vi "read channel page lecroy.vi"(0 "VISA in":refnum<visa-resource-name>, 5 "Crate":i32, 7 "page":i32, 11 "error in":errorcluster) -> (4 "VISA out":refnum<visa-resource-name>, 6 "Array":T1[](array[typedef]) {"Vfile (V)" format="%.1f V"; "Vswmax (V)" format="%#_g V"; "Iset (A)" format="%.2pA"; "Imon (A)" format="%.2pA"; "Vset (V)" format="%#_g V"; "Vmon (V)" format="%.1f V"}, 8 "New Channels":T1[](array[typedef]) {"Vfile (V)" format="%.1f V"; "Vswmax (V)" format="%#_g V"; "Iset (A)" format="%.2pA"; "Imon (A)" format="%.2pA"; "Vset (V)" format="%#_g V"; "Vmon (V)" format="%.1f V"}, 10 "Start Index in ACTIVE":i32, 15 "error out":errorcluster)   [LabVIEW 2018]
uses:
  channel_cluster.ctl
  Tom Shaw/Lecroy Control/HV Documentation and Software for Testing/SubVIs/General_lecroy_command.ctl
  channel.ctl
  CAEN globals.vi
  <userlib>/_OpenG.lib/array/array.llb/Filter 1D Array with Scalar (I32)__ogtk.vi
panel:
  # "Press Ctrl+M to open the master for edit"
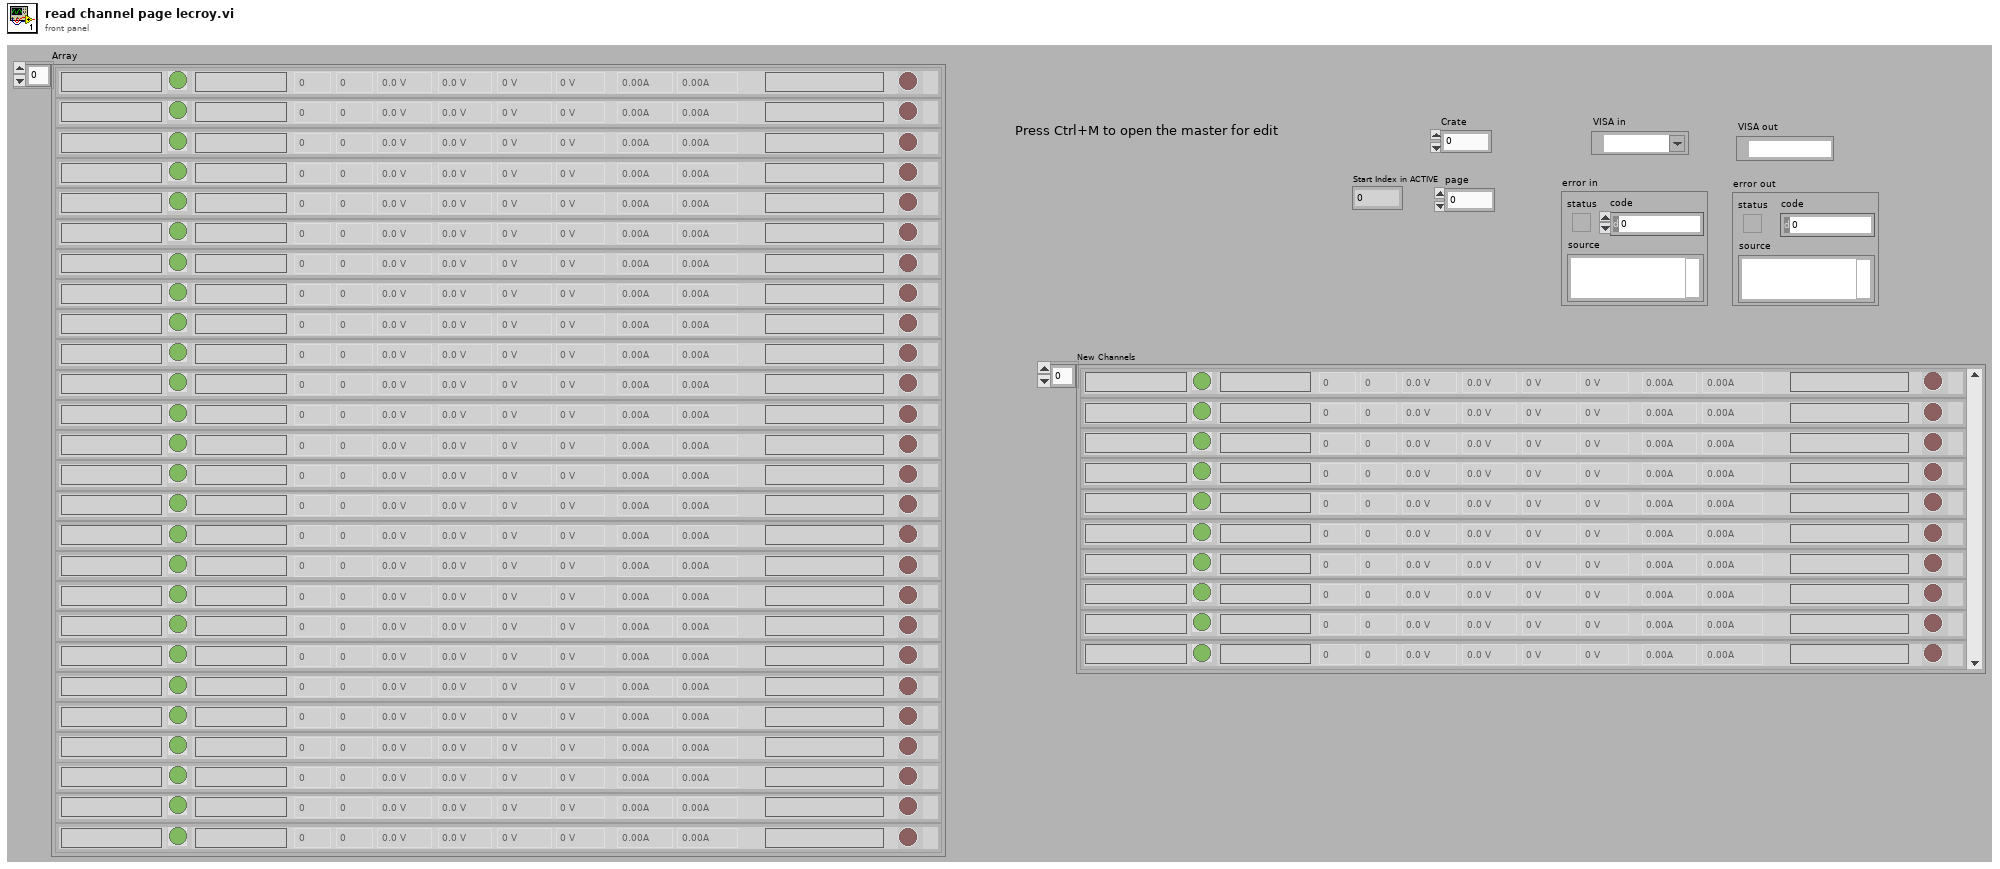
[diagram p1: front panel]
types:
  T1 = typedef "channel_cluster.ctl" = cluster{"Channel Name":string, "Crate":i32, "Card Type":string, "Card":i32, "Channel":i32, "Status Icon":picture, "Vmon (V)":dbl, "Vset (V)":dbl, "Imon (A)":dbl, "Iset (A)":dbl, "Timestamp":string, "ON/OFF":bool, "Status":string, "Vswmax (V)":dbl, "Flag":bool, "Vfile (V)":dbl, "Error Logged":bool[], "enable_file":bool}
  T2 = enum16{"Monitor", "Demand", "Backup", "All", "None"}
  T3 = typedef "crate.ctl" = cluster{"CAENet Address":i32, "Crate Model":string, "Firmware Version":string, "Crate Map":T4[], "Total Channels":i32}
  T4 = typedef "card.ctl" = cluster{"Slot Number":i32, "Card Model":string, "Num Channels":i32, "Polarity":string, "Vmax":dbl, "Imax":dbl, "Revision":string}
  T5 = typedef "General_lecroy_command.ctl" = string
  T6 = typedef "channel.ctl" = cluster{" Card.Channel":dbl, "Crate":i32}
  T7 = cluster{"Group Name":string, "Channels in Group":T6[]}[]
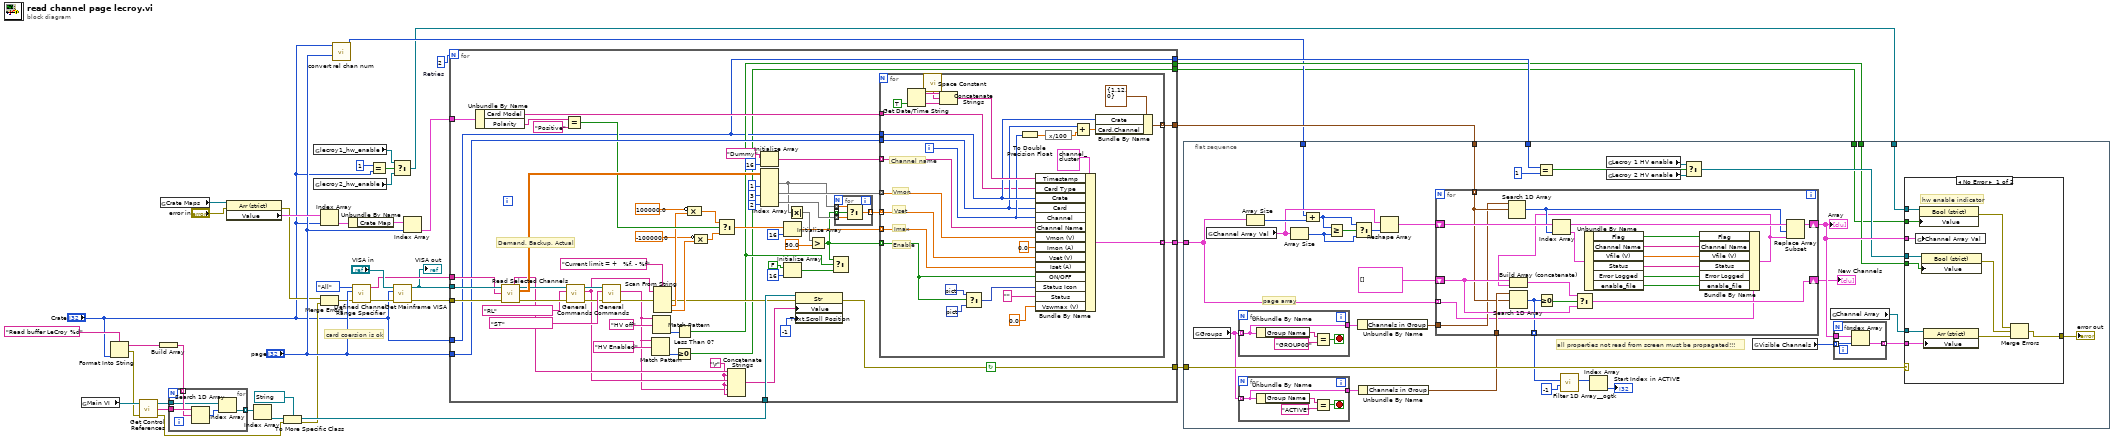
[diagram p0: block diagram]
diagram:
  w41 = 2  # Retries
  # "card coersion is ok"
  n1 = global read "CAEN globals.vi" "Main VI"() -> (w22:refnum<vi>)
  n2 = Format Into String(format string="Read buffer LeCroy %d" ("Label.Text"), "Crate") -> (resulting string=w12:string, error out=w13:errorcluster)  [unwired: 2 in]
  n3 = call "Get Control References.vi"("error in"=w13, "This vi"=w22) -> ("error out"=w19:errorcluster, "Control Names"=w23:string[], "Controls[]"=w24:refnum<vi>[])  [unwired: 1 in]
  n4 = Build Array(w12) -> (w14:string[])
  n5 = global read "CAEN globals.vi" "Crate Maps"() -> (w40:refnum<vi>)
  n6 = for {
    tunnel: w23 -> [w47]
    tunnel: w14 -> [w46] mode=indexing
    tunnel: w24 -> [w45]
    tunnel: [w44] -> w25 mode=indexing
    n7 = Search 1D Array(1D array=w47, element=w46) -> (index of element=w43:i32)  [unwired: 1 in]
    n8 = Index Array(array=w45, index=w43) -> (element=w44:refnum<vi>)
  }
  n9 = property class="Arr (strict)"(reference=w40, error in="error in") -> (error out=w17:errorcluster, "Value"=w30:T3[])  [unwired: 1 out]
  n10 = Index Array(array=w25) -> (element=w20:refnum<vi>)  [unwired: 1 in]
  n11 = To More Specific Class(target class=refnum<vi> refnum ("s? t:f"), reference=w20, error in=w19) -> (specific class reference=w18:refnum<vi>, error out=w16:errorcluster)
  n12 = global read "CAEN globals.vi" "lecroy1_hw_enable"() -> (w4:refnum<vi>)
  n13 = global read "CAEN globals.vi" "lecroy2_hw_enable"() -> (w3:refnum<vi>)
  n14 = Merge Errors(w17, w16) -> (w15:errorcluster)
  n15 = Index Array(array=w30, index="Crate") -> (element=w29:T3)
  n16 = call "convert rel chan num.vi"("Card"="page", "Crate"="Crate") -> ("Absolute index"=w8:i32)  [unwired: 6 in, 3 out]
  n17 = Unbundle By Name(w29) -> ("Crate Map"=w28:T4[])
  n18 = call "Defined Channel Range Specifier.vi"("error in"=w15, "Card"="page", "Buffer"=T2."All") -> ("error out"=w35:errorcluster, "Channel Range"=w34:string)  [unwired: 7 in]
  n19 = Equal?(x=1, y="Crate") -> (x = y?=w7:bool)
  n20 = Select(t=w4, s=w7, f=w3) -> (s? t:f=w2:refnum<vi>)
  n21 = call "Get Mainframe VISA.vi"("Error In"=w35, "Crate"="Crate", "VISA In"="VISA in") -> ("Error Out"=w37:errorcluster, "VISA out"=w32:refnum<visa-resource-name>)  [unwired: 6 in, 1 out]
  "VISA out" <- w32
  n22 = Index Array(array=w28, index="page") -> (element=w27:T4)
  n23 = for {
    N: w41 -> [_]
    tunnel: w32 -> [w106]
    tunnel: [w108] -> w31
    tunnel: w37 -> [w105]
    tunnel: [w61] -> w42
    tunnel: [w107] -> w39
    tunnel: w34 -> [w104]
    tunnel: "Crate" -> [w51]
    tunnel: "page" -> [w89]
    tunnel: w27 -> [w81]
    tunnel: w18 -> [w67]
    tunnel: [w56] -> w9
    tunnel: [w51] -> w10
    tunnel: [w50] -> w1
    stop <- w61 continue-if-true
    w63 = "\r"
    # "Demand, Backup, Actual"
    n24 = Unbundle By Name(w81) -> ("Card Model"=w87:string, "Polarity"=w86:string)
    n25 = call "Read Selected Channels.vi"("VISA in"=w106, "C##,##DO###"=w104, "error in"=w105) -> ("Final Output"=w66:string, "VISA out"=w98:refnum<visa-resource-name>, "Channel Array"=w103:dbl[][], "error out"=w99:errorcluster)  [unwired: 6 in, 3 out]
    n26 = Equal?(x=w86, y="Positive") -> (x = y?=w82:bool)
    n27 = call "General Commands.vi"("error in"=w99, "Action"=T5 "RL", "VISA in"=w98) -> ("error out"=w84:errorcluster, "result string"=w65:string, "VISA out"=w94:refnum<visa-resource-name>)  [unwired: 6 in]
    n28 = call "General Commands.vi"("error in"=w84, "Action"=T5 "ST", "VISA in"=w94) -> ("error out"=w83:errorcluster, "result string"=w48:string)  [unwired: 6 in, 1 out]
    n29 = Match Pattern(string=w48, regular expression="HV Enabled") -> (offset past match=w52:i32)  [unwired: 1 in, 3 out]
    n30 = Match Pattern(string=w48, regular expression="HV off") -> (offset past match=w78:i32)  [unwired: 1 in, 3 out]
    n31 = Scan From String(format string="Current limit = +   %f, - %f", input string=w65, error in=w83) -> (error out=w62:errorcluster, output 1=w74:dbl, output 2=w69:dbl)  [unwired: 3 in, 2 out]
    n32 = Greater Or Equal To 0?(x=w52) -> (x >= 0?=w50:bool)
    n33 = Less Than 0?(x=w78) -> (x < 0?=w56:bool)
    n34 = Compound Arithmetic op=MULTIPLY(invert 100000.0 ("value"), w74) -> (w73:dbl)
    n35 = Compound Arithmetic op=MULTIPLY(invert -100000.0 ("value"), w69) -> (w71:dbl)
    n36 = Select(t=w73, s=w82, f=w71) -> (s? t:f=w80:dbl)
    n37 = Concatenate Strings(w66, w63, w65, w63, w48, w63) -> (w64:string)
    n38 = Initialize Array("Dummy" ("regular expression"), 16 ("dimension size")) -> (w76:string[])
    n39 = Index Array(array=w103, index (col) #1=1 ("disabled index (col)"), index (col) #2=3 ("disabled index (col)"), index (col) #3=2 ("disabled index (col)")) -> (element #1=w54:dbl[], element #2=w100:dbl[], element #3=w58:dbl[])  [unwired: 3 in]
    n40 = Initialize Array(w80, 16 ("dimension size")) -> (w95:dbl[])
    n41 = Initialize Array(FALSE ("x = y?"), 16 ("dimension size")) -> (w90:bool[])
    n42 = Absolute Value(x=w54) -> (abs(x)=w53:dbl[])
    n43 = property class="Str"(reference=w67, error in=w62, "Value"=w64, "Text.Scroll Position"=-1) -> (error out=w61:errorcluster)  [unwired: 1 out]
    n44 = Greater?(x=w53, y=50.0 ("value")) -> (0:w57:bool[])
    n45 = Select(t=w57, s=w56, f=w90) -> ()  [unwired: 1 out]
    n46 = for {
      tunnel: [w112] -> w59 mode=indexing
      tunnel: w57 -> [w111] mode=indexing
      tunnel: w54 -> [w110] mode=indexing
      tunnel: w58 -> [w109] mode=indexing
      n47 = Select(t=w110, s=w111, f=w109) -> (s? t:f=w112:dbl)
    }
    n48 = for {
      tunnel: w76 -> [w129] mode=indexing
      tunnel: w100 -> [w119] mode=indexing
      tunnel: w59 -> [w120] mode=indexing
      tunnel: w95 -> [w121] mode=indexing
      tunnel: w57 -> [w122] mode=indexing
      tunnel: [w135] -> w108 mode=indexing
      tunnel: w51 -> [w126]
      tunnel: [w125] -> w107 mode=indexing
      tunnel: w89 -> [w123]
      tunnel: w87 -> [w114]
      i -> [w124]
      # "Channel name"
      # "Enable"
      # "Imax"
      # "Vset"
      # "Vmon"
      n49 = Get Date/Time String(want seconds? (F)=TRUE) -> (date string=w139:string, time string=w138:string)  [unwired: 2 in]
      n50 = call <vilib>:"Space Constant.vi"() -> ("String"=w137:string)
      n51 = Concatenate Strings(w139, w137, w138) -> (w130:string)
      n52 = Select(t=picture bytes[830] ("Status Icon 2"), s=w122, f=picture bytes[830] ("new picture 2")) -> (s? t:f=w134:picture)
      n53 = To Double Precision Float(number=w124) -> (double precision float=w132:dbl)
      n54 = Bundle By Name(cluster=T1 {"Channel Name"="", "Crate"=0, "Card Type"="", "Card"=0, "Channel"=0, "Status Icon"=bytes[0], "Vmon (V)"=0.0, "Vset (V)"=0.0, "Imon (A)"=0.0, "Iset (A)"=0.0, "Timestamp"="", "ON/OFF"=FALSE, "Status"="", "Vswmax (V)"=0.0, "Flag"=FALSE, "Vfile (V)"=0.0, "Error Logged"=[], "enable_file"=FALSE} ("Channel cluster"), "Timestamp"=w130, "Card Type"=w114, "Crate"=w126, "Card"=w123, "Channel"=w124, "Channel Name"=w129, "Vmon (V)"=w119, "Imon (A)"=0.0 ("element"), "Vset (V)"=w120, "Iset (A)"=w121, "ON/OFF"=w122, "Status Icon"=w134, "Status"="" ("y"), "Vswmax (V)"=0.0 ("number")) -> (w135:T1)
      n55 = expression code="x/100"(w132) -> (w133:dbl)
      n56 = Add(x=w123, y=w133) -> (x+y=w127:dbl)
      n57 = Bundle By Name(cluster=T6 {" Card.Channel"=1.12, "Crate"=0} ("Cluster"), "Crate"=w126, "Card.Channel"=w127) -> (w125:T6)
    }
  }
  n58 = flat-sequence {
    tunnel: w42 -> [w164]
    tunnel: w39 -> [w162]
    tunnel: w31 -> [w160]
    tunnel: w8 -> [w159]
    tunnel: w10 -> [w155]
    tunnel: w9 -> [w152]
    tunnel: w2 -> [w141]
    tunnel: w1 -> [w140]
    frame #0 {
      # "all properties not read from screen must be propagated!!!"
      # "page array"
      n59 = global read "CAEN globals.vi" "Groups"() -> (w150:T7)
      n60 = global read "CAEN globals.vi" "Channel Array Val"() -> (w165:T1[])
      n61 = for {
        tunnel: w150 -> [w181] mode=indexing
        tunnel: [w181] -> w161
        stop <- w180 stop-if-true
        n62 = Unbundle By Name(w181) -> ("Group Name"=w183:string)
        n63 = Equal?(x=w183, y="GROUP00" ("Group Name")) -> (x = y?=w180:bool)
      }
      n64 = for {
        tunnel: w150 -> [w177] mode=indexing
        tunnel: [w177] -> w151
        stop <- w176 stop-if-true
        n65 = Unbundle By Name(w177) -> ("Group Name"=w179:string)
        n66 = Equal?(x=w179, y="ACTIVE" ("Group Name")) -> (x = y?=w176:bool)
      }
      n67 = Array Size(array=w160) -> (size(s)=w170:i32)
      n68 = Array Size(array=w165) -> (size(s)=w174:i32)
      n69 = Compound Arithmetic op=ADD(w159, w170) -> (w171:i32)
      n70 = Greater Or Equal?(x=w171, y=w174) -> (x >= y?=w175:bool)
      n71 = Select(t=w171, s=w175, f=w174) -> (s? t:f=w173:i32)
      n72 = Unbundle By Name(w161) -> ("Channels in Group"=w146:T6[])
      n73 = Unbundle By Name(w151) -> ("Channels in Group"=w149:T6[])
      n74 = Reshape Array(w165, w173) -> (w172:T1[])
      n75 = for {
        tunnel: w160 -> [w200] mode=indexing
        shift-right: [w215] -> w167
        shift-left: w172 -> [w214]
        tunnel: w162 -> [w202] mode=indexing
        tunnel: w149 -> [w207]
        shift-right: [w204] -> w148
        shift-left: T1[] [] -> [w203]
        tunnel: w146 -> [w201]
        tunnel: [w197] -> w145 mode=indexing
        n76 = Search 1D Array(1D array=w201, element=w202) -> (index of element=w213:i32)  [unwired: 1 in]
        n77 = Search 1D Array(1D array=w207, element=w202) -> (index of element=w197:i32)  [unwired: 1 in]
        n78 = Greater Or Equal To 0?(x=w197) -> (x >= 0?=w205:bool)
        n79 = Index Array(array=w214, index=w213) -> (element=w212:T1)
        n80 = Unbundle By Name(w212) -> ("Flag"=w211:bool, "Channel Name"=w210:string, "Vfile (V)"=w209:dbl, "Status"=w208:string, "Error Logged"=w198:bool[], "enable_file"=w196:bool)
        n81 = Bundle By Name(cluster=w200, "Flag"=w211, "Channel Name"=w210, "Vfile (V)"=w209, "Status"=w208, "Error Logged"=w198, "enable_file"=w196) -> (w199:T1)
        n82 = Build Array (concatenate)(w203, w199) -> (w206:T1[])
        n83 = Select(t=w206, s=w205, f=w203) -> (s? t:f=w204:T1[])
        n84 = Replace Array Subset(array=w214, new element=w199, index=w213) -> (w215:T1[])
      }
      "Array" <- w167
      "New Channels" <- w148
      n85 = Equal?(x=w155, y=1) -> (x = y?=w153:bool)
      n86 = call-poly <userlib>:"Filter 1D Array__ogtk.vi"("items to filter"=-1 ("Numeric"), "array"=w145) -> ("filtered array"=w143:i32[])  [unwired: 4 in, 1 out]
      n87 = Index Array(array=w143) -> (element=→"Start Index in ACTIVE":i32)  [unwired: 1 in]
      n88 = global read "CAEN globals.vi" "Lecroy 1 HV enable"() -> (w158:refnum<vi>)
      n89 = global read "CAEN globals.vi" "Lecroy 2 HV enable"() -> (w157:refnum<vi>)
      n90 = Select(t=w158, s=w153, f=w157) -> (s? t:f=w156:refnum<vi>)
      n91 = global read "CAEN globals.vi" "Visible Channels"() -> (w168:i32[])
      n92 = global read "CAEN globals.vi" "Channel Array"() -> (w169:refnum<vi>)
      n93 = for {
        tunnel: w168 -> [w217] mode=indexing
        tunnel: w167 -> [w218]
        tunnel: [w216] -> w166 mode=indexing
        n94 = Index Array(array=w218, index=w217) -> (element=w216:T1)
      }
      n95 = case shown="No Error" w164 {
        selector: w164 -> [_ w195]
        tunnel: w169 -> [w194 _]
        tunnel: w167 -> [w193 _]
        tunnel: w166 -> [w192 _]
        tunnel: [w190 w195] -> w163
        tunnel: w156 -> [w188 _]
        tunnel: w152 -> [w187 _]
        tunnel: w141 -> [w186 _]
        tunnel: w140 -> [w184 _]
        frame No Error {
          # "hw enable indicator"
          n96 = global write "CAEN globals.vi" "Channel Array Val"(w193) -> ()
          n97 = property class="Bool (strict)"(reference=w186, "Value"=w184) -> (error out=w185:errorcluster)  [unwired: 1 in, 1 out]
          n98 = property class="Bool (strict)"(reference=w188, "Value"=w187) -> (error out=w189:errorcluster)  [unwired: 1 in, 1 out]
          n99 = property class="Arr (strict)"(reference=w194, "Value"=w192) -> (error out=w191:errorcluster)  [unwired: 1 in, 1 out]
          n100 = Merge Errors(w185, w189, w191) -> (w190:errorcluster)
        }
        frame Error {
        }
      }
      "error out" <- w163
    }
  }
